vi "Select Projectile Type.vi"(2 "projectileWeight":string) -> (0 "projectileTypes":string[](array[string]))   [LabVIEW 2010]
panel:
  out "error OUT":errorcluster
  in  "error IN":errorcluster
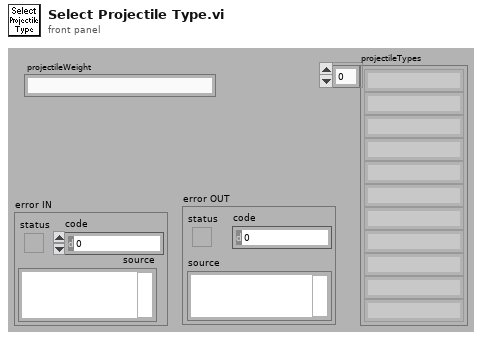
[diagram p1: front panel]
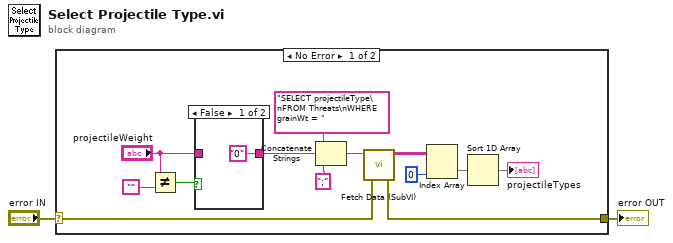
[diagram p0: block diagram]
diagram:
  n1 = case shown="No Error" "error IN" {
    selector: "error IN" -> [w4 w18]
    tunnel: [w3 w18] -> w1
    frame No Error {
      n2 = Not Equal?(x="projectileWeight", y="") -> (x != y?=w7:bool)
      n3 = case shown="False" w7 {
        tunnel: ["0" ("projectileWeight") w17] -> w5
        tunnel: "projectileWeight" -> [_ w17]
        frame False {
        }
        frame True {
        }
      }
      n4 = Concatenate Strings("SELECT projectileType\nFROM Threats\nWHERE grainWt = ", w5, ";" ("string")) -> (w11:string)
      n5 = call "Fetch Data (SubVI).vi"("error IN"=w4, "query string"=w11) -> ("error OUT"=w3:errorcluster, "recordset data"=w15:string[][])  [unwired: 4 out]
      n6 = Index Array(array=w15, index (col)=0 ("disabled index (col)")) -> (element=w10:string[])  [unwired: 1 in]
      n7 = Sort 1D Array(array=w10) -> (sorted array=→"projectileTypes":string[])
    }
    frame Error {
    }
  }
  "error OUT" <- w1
